vi "Launch Custom Device XML Configuration Tool.vi"   [LabVIEW 2019]
uses:
  Support/Configuration Tool Main.vi
  Support/Configuration Tool.lvlib
panel:
  # "Loading Custom Device XML Configuration Tool"
types:
  T1 = enum32{"Invalid", "Standard", "Closed", "Hidden", "Minimized", "Maximized"}
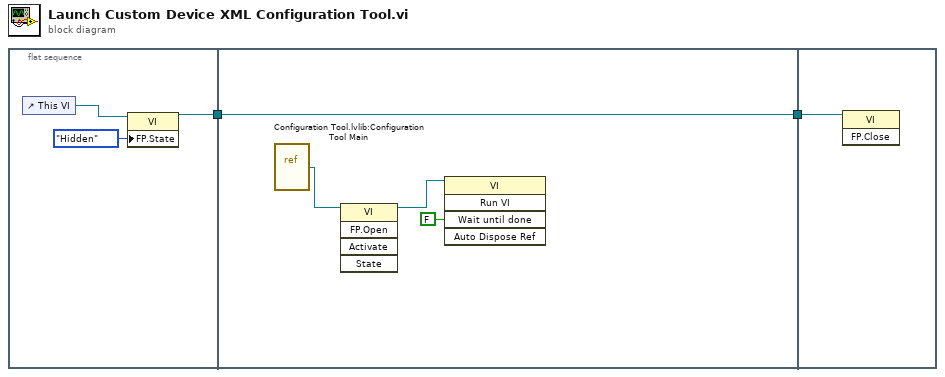
[diagram p0: block diagram]
diagram:
  n1 = flat-sequence {
    tunnel: [w4] -> w2
    tunnel: w2 -> [w9]
    tunnel: [w9] -> w1
    tunnel: w1 -> [w10]
    frame #0 {
      n2 = control-ref of="This VI"() -> (w3:refnum<vi>)
      n3 = property class="VI"(reference=w3, "FP.State"=T1."Hidden" ("Front Panel Window:State")) -> (reference out=w4:refnum<vi>)  [unwired: 1 in, 1 out]
    }
    frame #1 {
      n4 = vi-ref "Configuration Tool.lvlib:Configuration Tool Main.vi"() -> (w8:refnum<vi>)
      n5 = invoke class="VI" method="FP.Open"(reference=w8) -> (reference out=w7:refnum<vi>)  [unwired: 4 in, 4 out]
      n6 = invoke class="VI" method="Run VI"(reference=w7, "Wait until done"=FALSE ("Wait Until Done")) -> ()  [unwired: 3 in, 5 out]
    }
    frame #2 {
      n7 = invoke class="VI" method="FP.Close"(reference=w10) -> ()  [unwired: 2 in, 3 out]
    }
  }
